vi "READ ARM ANGLE TABLE.vi"(0 "file path (dialog if empty)":path=path "FRC2867_2022_robot_arm_data.txt", 5 "error in (no error)":errorcluster) -> (14 "shuttle X pos":dbl[](array[numeric]), 15 "arm angle to horiz":dbl[](array[numeric]), 17 "LIMIT ht":dbl[](array[numeric]), 18 "LIMIT ht HANGAR":dbl[](array[numeric]), 19 "error out":errorcluster)   [LabVIEW 2020]
uses:
  <vilib>/Analysis/6fits.llb/Curve Fitting Criteria.ctl
  <vilib>/Utility/file.llb/Read Delimited Spreadsheet (DBL).vi
  <vilib>/Rock Robotics/Network Tables/NT Write Numeric Array.vi
  Robot Global Data.vi
  <vilib>/Analysis/NI_AALPro.lvlib
panel:
  in  "arm angle table":T1
  in  "String":string="/home/lvuser/natinst/bin/data"
  out "new file path (Not A Path if cancelled) 2":path
  out "folder names":string[](array[string])
  out "filenames":string[](array[string])
  out "path out":path
  out "Target":string
  out "error":i32
  out "interpolation error":dbl format="%0.2f"
  out "interpolation value":dbl format="%0.2f"
  in  "X value to find":dbl
  out "file directory":path
  out "slope for X<0":dbl
  out "slope for X>0":dbl
  out "intercept":dbl
  out "slope":dbl
  out "new file path (Not A Path if cancelled)":path
  out "XY Graph":cluster{dbl[], dbl[]}[](graph)
  out "size(s)":i32[](array[numeric])
  out "all rows":dbl[][](array[numeric])
  # "intercept for both is 90 deg"
  # "line fit:"
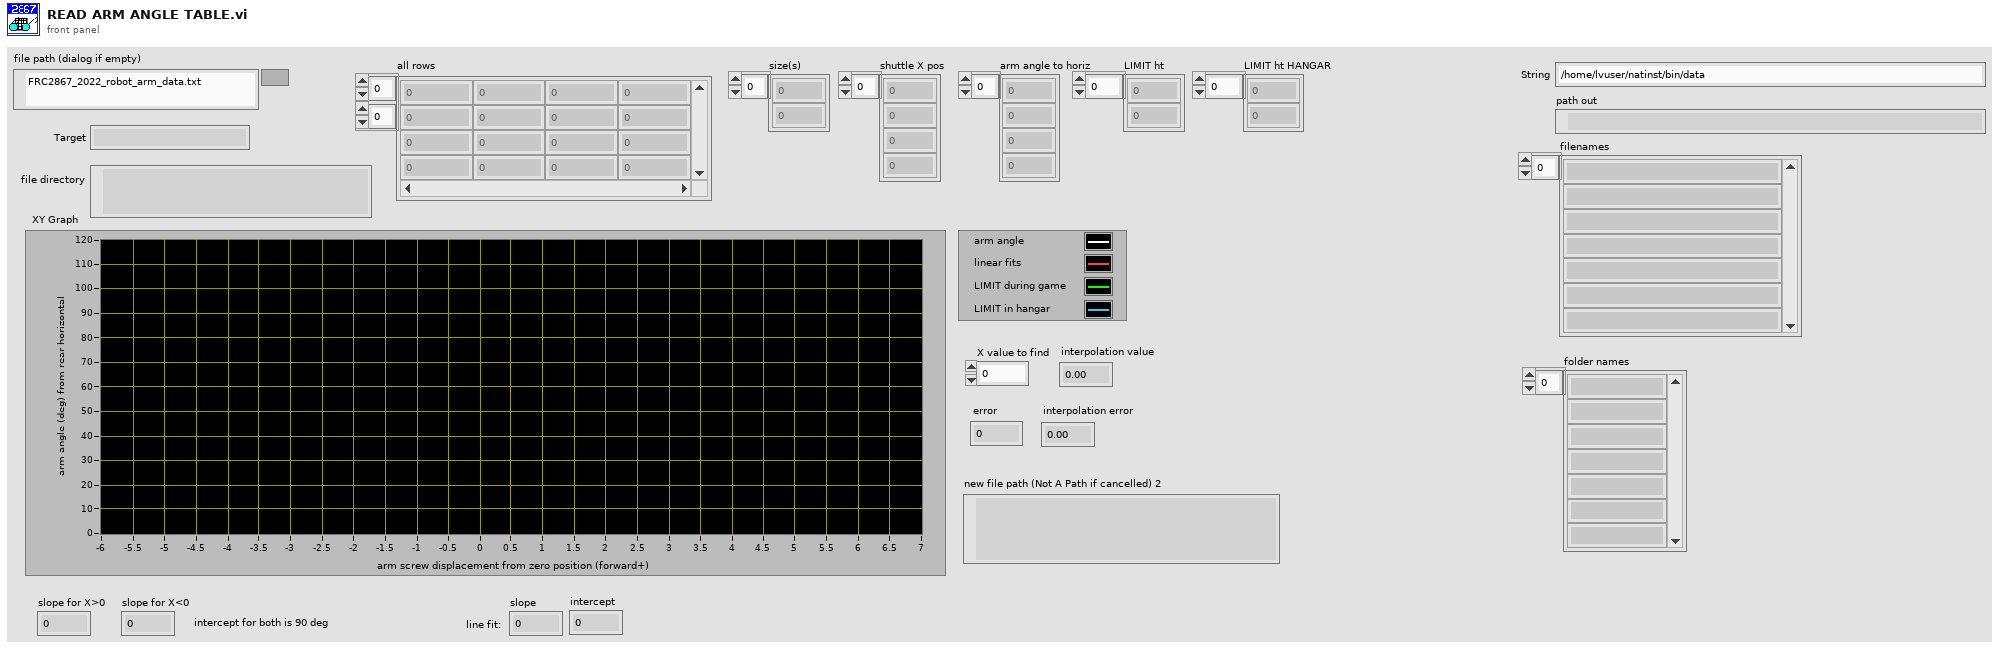
[diagram p1: front panel]
types:
  T1 = cluster{"X pos (in)":dbl[], "arm angle (deg)":dbl[], "ht LIMIT (in)":dbl[], "ht HANGAR (in)":dbl[]}
  T2 = typedef "NI_AALPro.lvlib/Curve Fitting Criteria.ctl" = u16
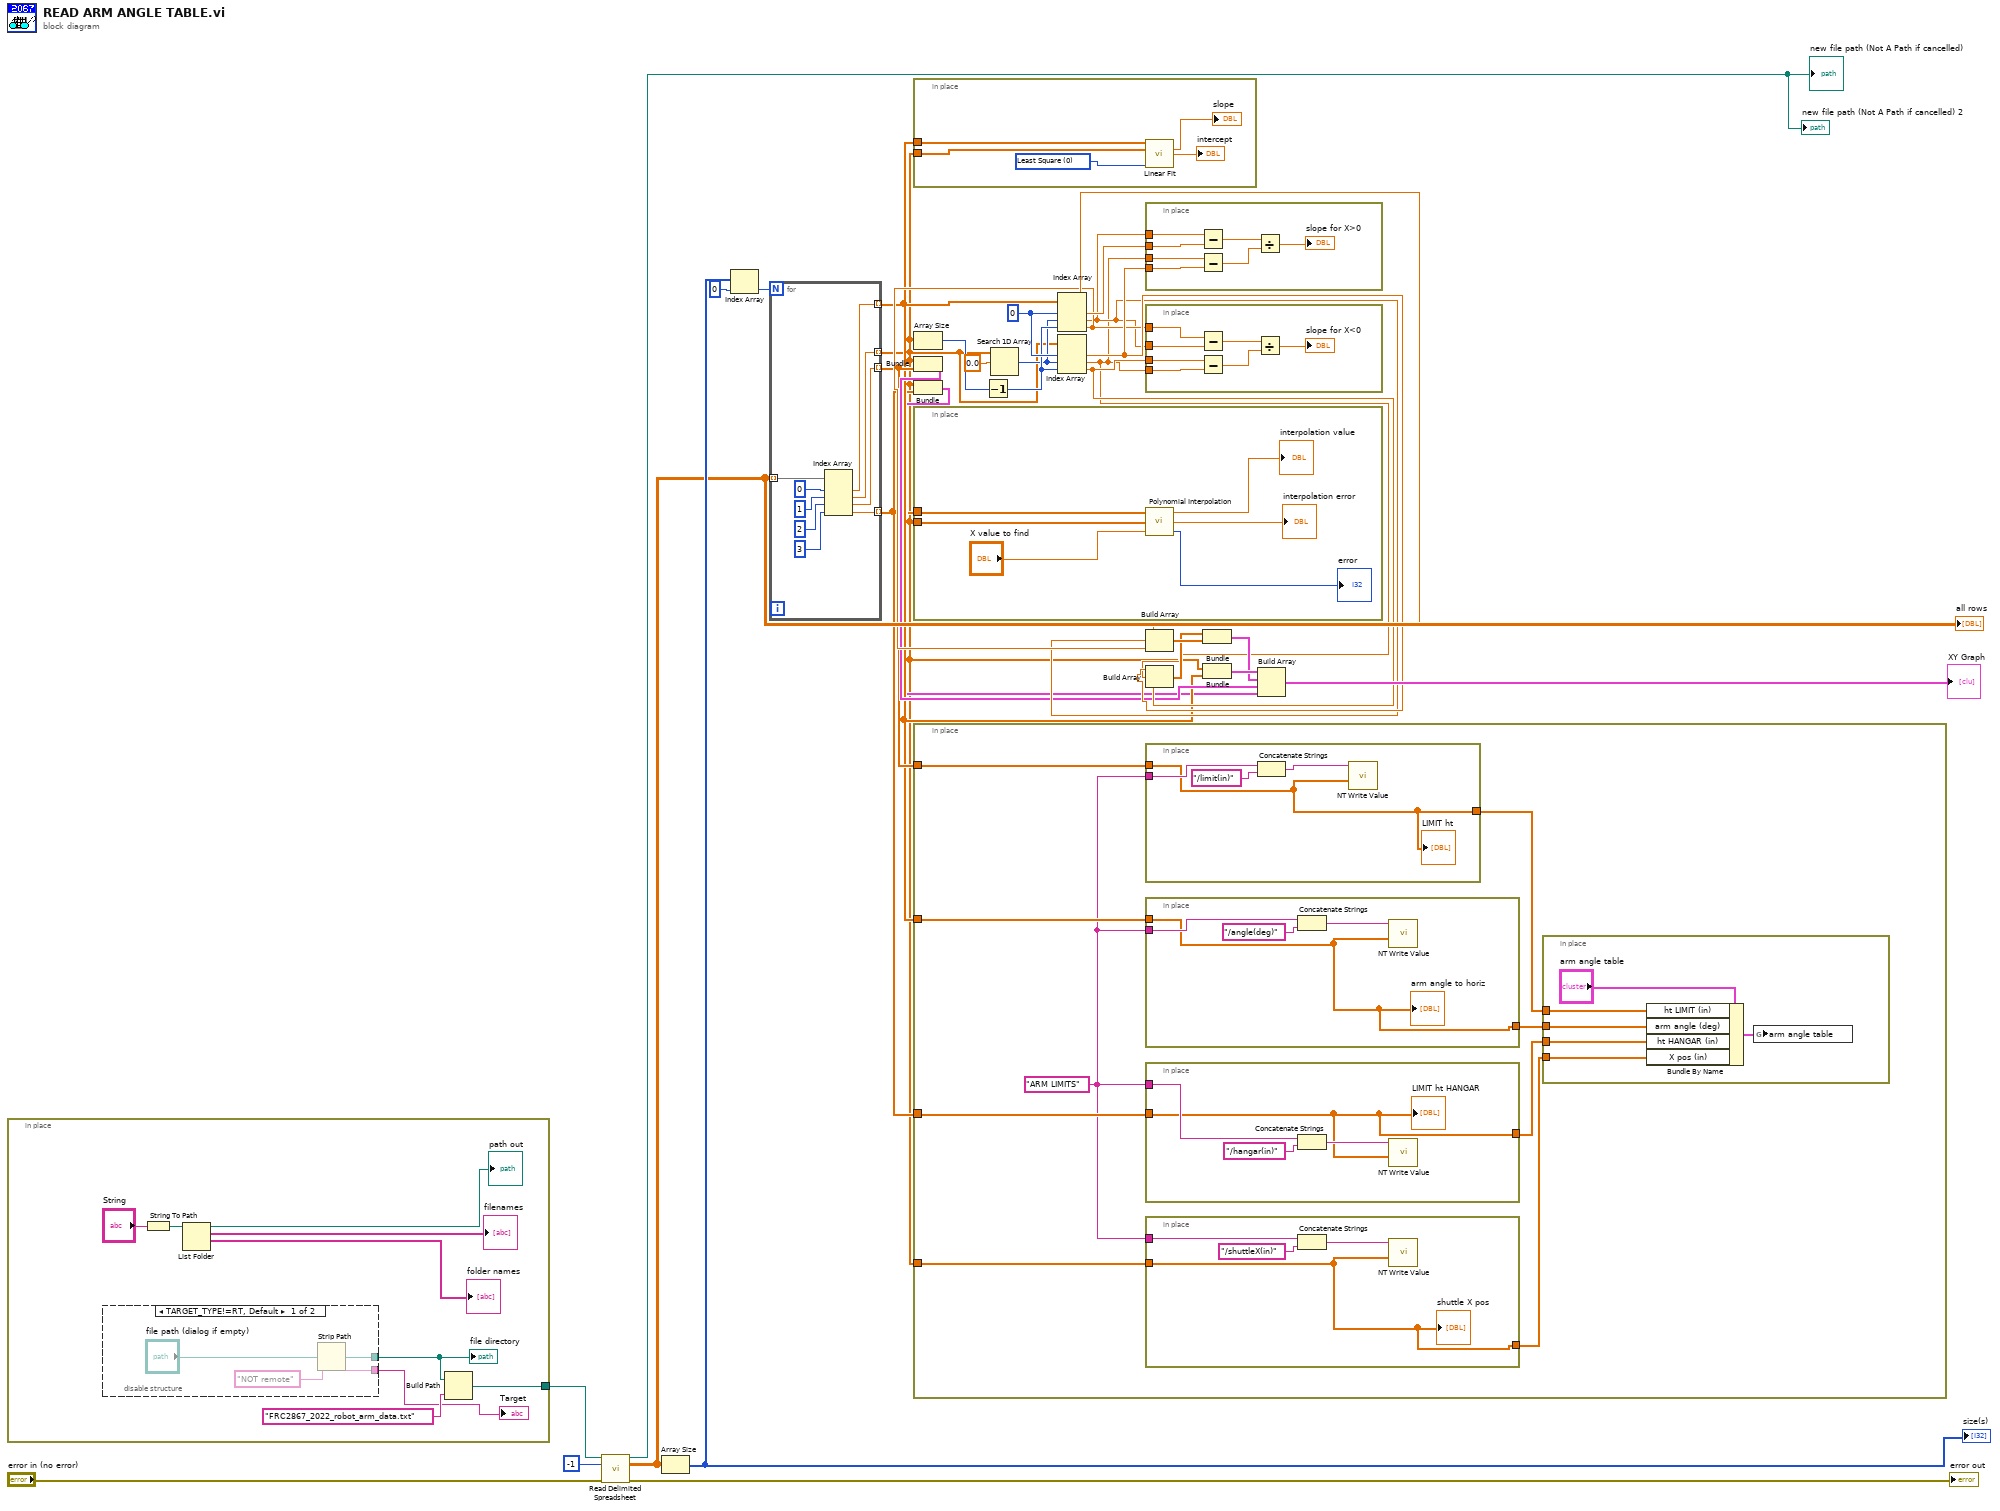
[diagram p0: block diagram]
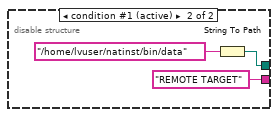
[diagram p2: hidden frame]
diagram:
  w20 = 0 ("index")
  n1 = in-place {
    in-place-border: [w40] -> w1
    n2 = disable-structure shown="TARGET_TYPE!=RT, Default" {
      disable-tunnel: [w41 w45] -> w34
      disable-tunnel: ["NOT remote" ("Target") "REMOTE TARGET" ("Target")] -> w38
      frame condition #0 {
        n3 = Strip Path(path="file path (dialog if empty)") -> (stripped path=w41:path)  [unwired: 1 out]
      }
      frame condition #1 (active) {
        n4 = String To Path(string="/home/lvuser/natinst/bin/data" ("String")) -> (path=w45:path)
      }
    }
    "file directory" <- w34
    "Target" <- w38
    n5 = String To Path(string="String") -> (path=w33:path)
    n6 = List Folder(path=w33) -> (path out=→"path out":path, filenames=→"filenames":string[], folder names=→"folder names":string[])  [unwired: 3 in, 1 out]
    n7 = Build Path(base path=w34, name or relative path="FRC2867_2022_robot_arm_data.txt" ("filename")) -> (appended path=w40:path)
  }
  n8 = call-poly <vilib>:"Read Delimited Spreadsheet.vi"("file path (dialog if empty)"=w1, "number of rows (all:-1)"=-1, "error in (no error)"="error in (no error)") -> ("new file path (Not A Path if cancelled)"=→"new file path (Not A Path if cancelled)" →"new file path (Not A Path if cancelled) 2":path, "all rows"=w27:dbl[][], "error out"=→"error out":errorcluster)  [unwired: 7 in, 3 out]
  "all rows" <- w27
  n9 = Array Size(array=w27) -> (size(s)=w30:i32[])
  "size(s)" <- w30
  n10 = Index Array(array=w30, index=0) -> (element=w28:i32)
  n11 = for {
    N: w28 -> [_]
    tunnel: w27 -> [w55] mode=indexing
    tunnel: [w54] -> w5 mode=indexing
    tunnel: [w53] -> w2 mode=indexing
    tunnel: [w48] -> w3 mode=indexing
    tunnel: [w47] -> w6 mode=indexing
    n12 = Index Array(array=w55, index #1=0 ("index"), index #2=1 ("index"), index #3=2 ("index"), index #4=3 ("index")) -> (element #1=w54:dbl, element #2=w53:dbl, element #3=w47:dbl, element #4=w48:dbl)
  }
  n13 = in-place {
    in-place-border: w5 -> [w60]
    in-place-border: w2 -> [w59]
    w58 = T2 0 items=["Least Square", "Least Absolute Residual", "Bisquare"] ("method")
    n14 = call <vilib>:"Linear Fit.vi"("Y"=w60, "X"=w59, "method"=w58) -> ("slope"=→"slope":dbl, "intercept"=→"intercept":dbl)  [unwired: 8 in, 3 out]
  }
  n15 = Array Size(array=w2) -> (size(s)=w21:i32)
  n16 = Bundle(w2, w6) -> (w7:cluster{dbl[], dbl[]})  [unwired: 1 in]
  n17 = Bundle(w2, w3) -> (w4:cluster{dbl[], dbl[]})  [unwired: 1 in]
  n18 = in-place {
    in-place-border: w3 -> [w66]
    in-place-border: w2 -> [w65]
    n19 = call <vilib>:"Polynomial Interpolation.vi"("x value"="X value to find", "X"=w65, "Y"=w66) -> ("error"=→"error":i32, "interpolation error"=→"interpolation error":dbl, "interpolation value"=→"interpolation value":dbl)
  }
  n20 = in-place {
    in-place-border: w6 -> [w74]
    in-place-border: w5 -> [w75]
    in-place-border: w3 -> [w73]
    in-place-border: w2 -> [w72]
    w71 = "ARM LIMITS"
    n21 = in-place {
      in-place-border: w74 -> [w94]
      in-place-border: w71 -> [w95]
      in-place-border: [w94] -> w67
      n22 = Concatenate Strings(w95, "/limit(in)" ("string")) -> (w96:string)
      n23 = call-poly <vilib>:"NT Write Value.vi"("Numeric Array"=w94, "Name"=w96) -> ()  [unwired: 9 in, 1 out]
      "LIMIT ht" <- w94
    }
    n24 = in-place {
      in-place-border: w75 -> [w86]
      in-place-border: w71 -> [w87]
      in-place-border: [w86] -> w68
      n25 = Concatenate Strings(w87, "/angle(deg)" ("string")) -> (w88:string)
      n26 = call-poly <vilib>:"NT Write Value.vi"("Numeric Array"=w86, "Name"=w88) -> ()  [unwired: 9 in, 1 out]
      "arm angle to horiz" <- w86
    }
    n27 = in-place {
      in-place-border: w73 -> [w82]
      in-place-border: w71 -> [w83]
      in-place-border: [w82] -> w69
      n28 = Concatenate Strings(w83, "/hangar(in)" ("string")) -> (w84:string)
      n29 = call-poly <vilib>:"NT Write Value.vi"("Numeric Array"=w82, "Name"=w84) -> ()  [unwired: 9 in, 1 out]
      "LIMIT ht HANGAR" <- w82
    }
    n30 = in-place {
      in-place-border: w72 -> [w90]
      in-place-border: w71 -> [w91]
      in-place-border: [w90] -> w70
      n31 = Concatenate Strings(w91, "/shuttleX(in)" ("string")) -> (w92:string)
      n32 = call-poly <vilib>:"NT Write Value.vi"("Numeric Array"=w90, "Name"=w92) -> ()  [unwired: 9 in, 1 out]
      "shuttle X pos" <- w90
    }
    n33 = in-place {
      in-place-border: w70 -> [w79]
      in-place-border: w69 -> [w78]
      in-place-border: w68 -> [w77]
      in-place-border: w67 -> [w76]
      n34 = Bundle By Name(cluster="arm angle table", "ht LIMIT (in)"=w76, "arm angle (deg)"=w77, "ht HANGAR (in)"=w78, "X pos (in)"=w79) -> (w81:T1)
      n35 = global write "Robot Global Data.vi" "arm angle table"(w81) -> ()
    }
  }
  n36 = Decrement(x=w21) -> (x-1=w15:i32)
  n37 = Search 1D Array(1D array=w2, element=0.0) -> (index of element=w14:i32)  [unwired: 1 in]
  n38 = Index Array(array=w5, index #1=w20, index #2=w14, index #3=w15) -> (element #1=w13:dbl, element #2=w10:dbl, element #3=w11:dbl)
  n39 = Index Array(array=w2, index #1=w20, index #2=w14, index #3=w15) -> (element #1=w12:dbl, element #2=w8:dbl, element #3=w9:dbl)
  n40 = in-place {
    in-place-border: w10 -> [w104]
    in-place-border: w13 -> [w103]
    in-place-border: w8 -> [w102]
    in-place-border: w12 -> [w101]
    n41 = Subtract(x=w104, y=w103) -> (x-y=w100:dbl)
    n42 = Subtract(x=w102, y=w101) -> (x-y=w99:dbl)
    n43 = Divide(x=w100, y=w99) -> (x/y=→"slope for X>0":dbl)
  }
  n44 = in-place {
    in-place-border: w11 -> [w111]
    in-place-border: w10 -> [w110]
    in-place-border: w9 -> [w109]
    in-place-border: w8 -> [w108]
    n45 = Subtract(x=w111, y=w110) -> (x-y=w107:dbl)
    n46 = Subtract(x=w109, y=w108) -> (x-y=w106:dbl)
    n47 = Divide(x=w107, y=w106) -> (x/y=→"slope for X<0":dbl)
  }
  n48 = Build Array(w13, w10, w11) -> (w18:dbl[])
  n49 = Build Array(w12, w8, w9) -> (w17:dbl[])
  n50 = Bundle(w17, w18) -> (w19:cluster{dbl[], dbl[]})  [unwired: 1 in]
  n51 = Bundle(w2, w5) -> (w26:cluster{dbl[], dbl[]})  [unwired: 1 in]
  n52 = Build Array(w26, w19, w7, w4) -> (→"XY Graph":cluster{dbl[], dbl[]}[])
